vi "test12.2-AsyncMessageWithReply_Event.vi"(8 "error in (no error)":errorcluster, 11 "TestCase in":refnum<class "testcase-CSMGlobalLog.lvclass">) -> (0 "error out":errorcluster, 3 "TestCase out":refnum<class "testcase-CSMGlobalLog.lvclass">)   [LabVIEW 2017, in "testcase-CSMGlobalLog.lvclass"]
uses:
  testcase-CSMGlobalLog.lvclass
  testcase-CSMGlobalLog.lvclass/testcase-CSMGlobalLog.ctl
  src/user.lib/_NEVSTOP/Communicable State Machine(CSM)/_Support/Typedef/_CSM_GlobalLog_MSG.ctl
  src/user.lib/_NEVSTOP/Communicable State Machine(CSM)/_Support/Typedef/_CSM_Response Source Message.ctl
  src/user.lib/_NEVSTOP/Communicable State Machine(CSM)/_Support/Typedef/_CSM_GlobalLog_MSG_TYPE.ctl
  c0dc643a-0362-49fc-99f4-5251266ba5a0.vi
  src/user.lib/_NEVSTOP/Communicable State Machine(CSM)/_Support/GlobalEvent/GEvt-Generate with Rule Check.vi
  src/user.lib/_NEVSTOP/Communicable State Machine(CSM)/AdvanceAPI/CSM - Convert Error to Argument.vi
  src/user.lib/_NEVSTOP/Communicable State Machine(CSM)/_Support/GlobalEvent/Cache-GEvt Refs.vi
  src/user.lib/_NEVSTOP/Communicable State Machine(CSM)/AdvanceAPI/CSM - Make String Arguments Safe.vi
  src/user.lib/_NEVSTOP/Communicable State Machine(CSM)/_Support/ChangeFlag/FlagInstance-GEvt Refs.vi
  src/user.lib/_NEVSTOP/Communicable State Machine(CSM)/AdvanceAPI/CSM - Keywords.vi
  src/user.lib/_NEVSTOP/Communicable State Machine(CSM)/_Support/ChangeFlag/ChangeFlag-Read.vi
  src/user.lib/_NEVSTOP/Communicable State Machine(CSM)/_Support/ChangeFlag/ChangeFlagDB.vi
  src/user.lib/_NEVSTOP/Communicable State Machine(CSM)/_Support/GlobalEvent/FGV-GlobalEventRef(lvlibp).vi
  src/user.lib/_NEVSTOP/Communicable State Machine(CSM)/_Support/GlobalEvent/FGV-GlobalEventQueues(lvlibp).vi
  src/user.lib/_NEVSTOP/Communicable State Machine(CSM)/_Support/GlobalEvent/GEvt-Valid Subscribers.vi
  src/user.lib/_NEVSTOP/Communicable State Machine(CSM)/_Support/GlobalEvent/LogFilter/LogFilter - Check.vi
  src/user.lib/_NEVSTOP/Communicable State Machine(CSM)/_Support/GlobalEvent/LogFilter/LogFilter.lvclass
  <vilib>/addons/_JKI Toolkits/VI Tester/TestCase.llb/TestCase.lvclass
  src/user.lib/_NEVSTOP/Communicable State Machine(CSM)/Communicable State Machine.lvlib
  C:/Program Files (x86)/National Instruments/LabVIEW 2017/vi.lib/addons/_JKI Toolkits/VI Tester/TestCase.llb/TestCase.lvclass
panel:
  out "String cache each loop":string
  out "LoopCount":i32
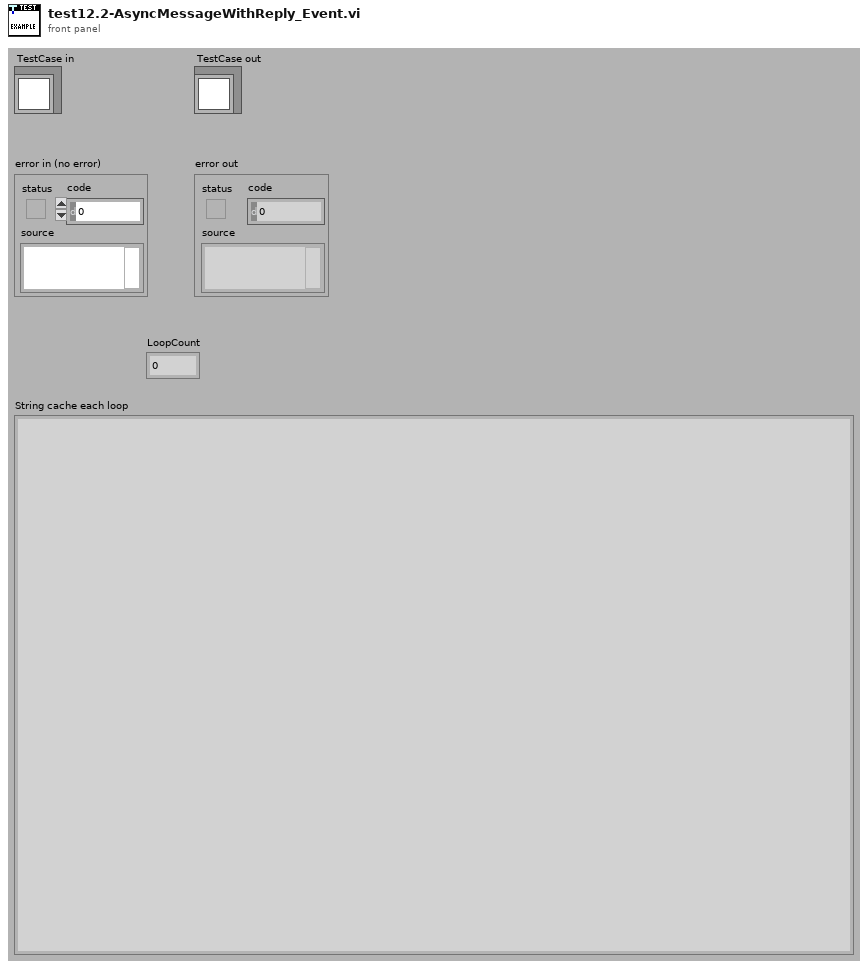
[diagram p1: front panel]
types:
  T1 = typedef "Communicable State Machine.lvlib/_CSM_GlobalLog_MSG.ctl" = cluster{"Name (\"\" to Use UUID)":string, "Current State":string, "Arguments":string, "Source Message":T2, "Source Module":string, "Complete(T)/Start(F)":bool, "LogType":T3, "Time Stamp":timestamp}
  T2 = typedef "Communicable State Machine.lvlib/_CSM_Response Source Message.ctl" = cluster{"‘State":string, "’Arguments":string, "’Error":errorcluster}
  T3 = typedef "Communicable State Machine.lvlib/_CSM_GlobalLog_MSG_TYPE.ctl" = enum16{"User Log", "State Change", "Status", "Interrupt", "Register", "Unregister", "Error Log", "Module Created", "Module Destroyed", "Async Message", "No-Rep Async Message", "Sync Message"}
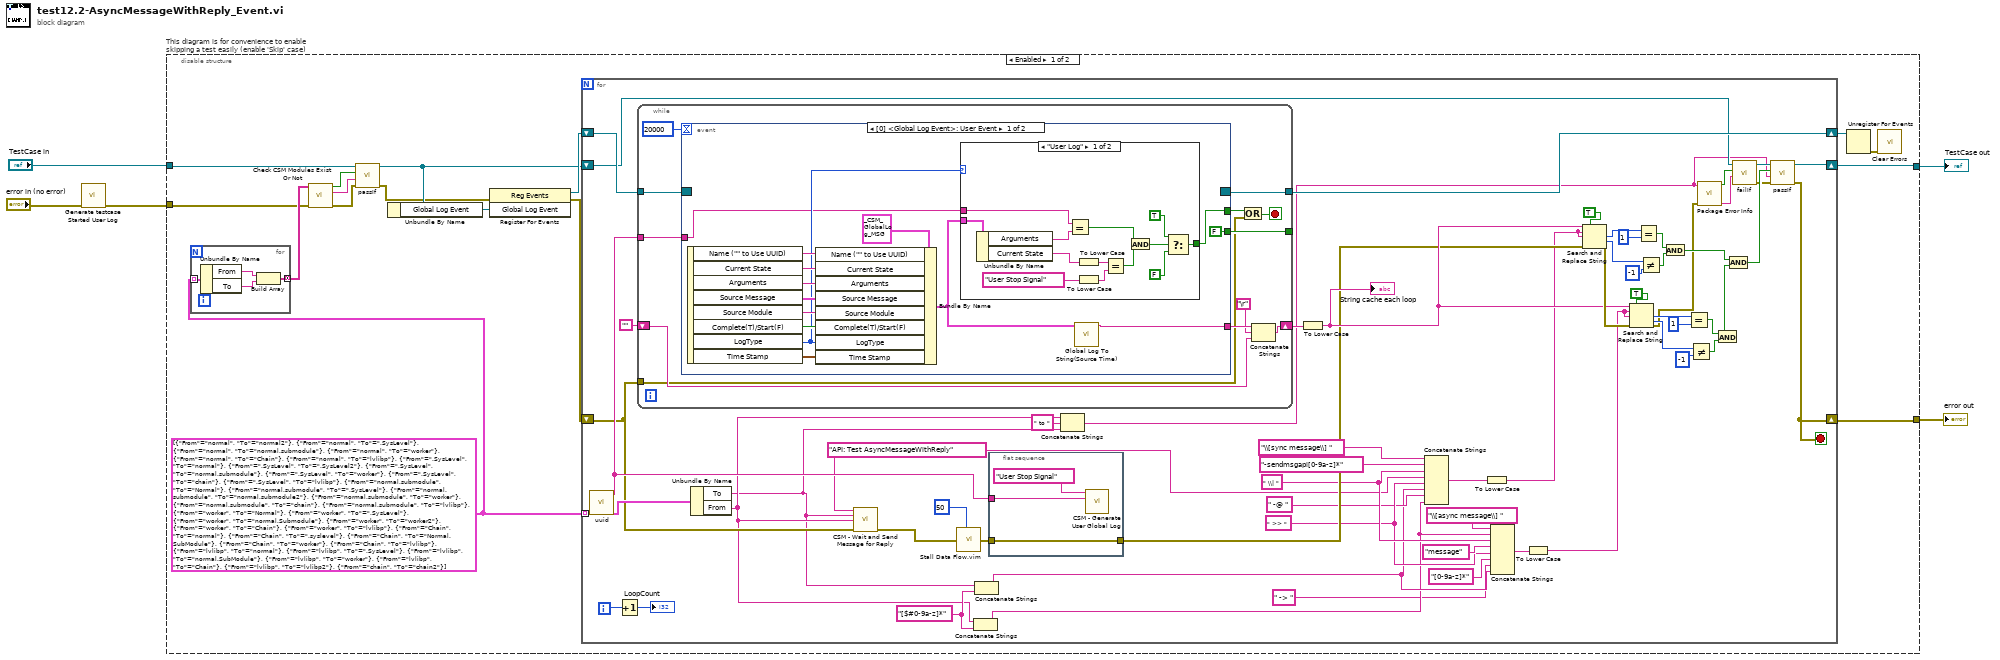
[diagram p0: block diagram]
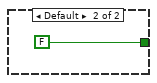
[diagram p2: hidden frame]
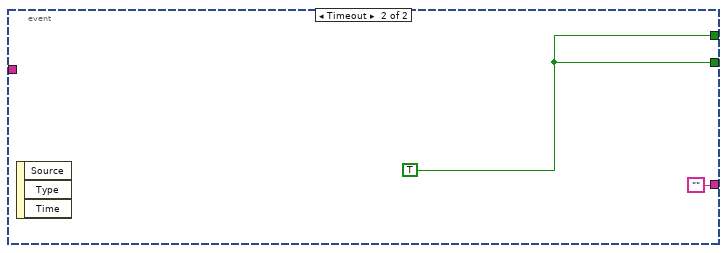
[diagram p3: hidden frame]
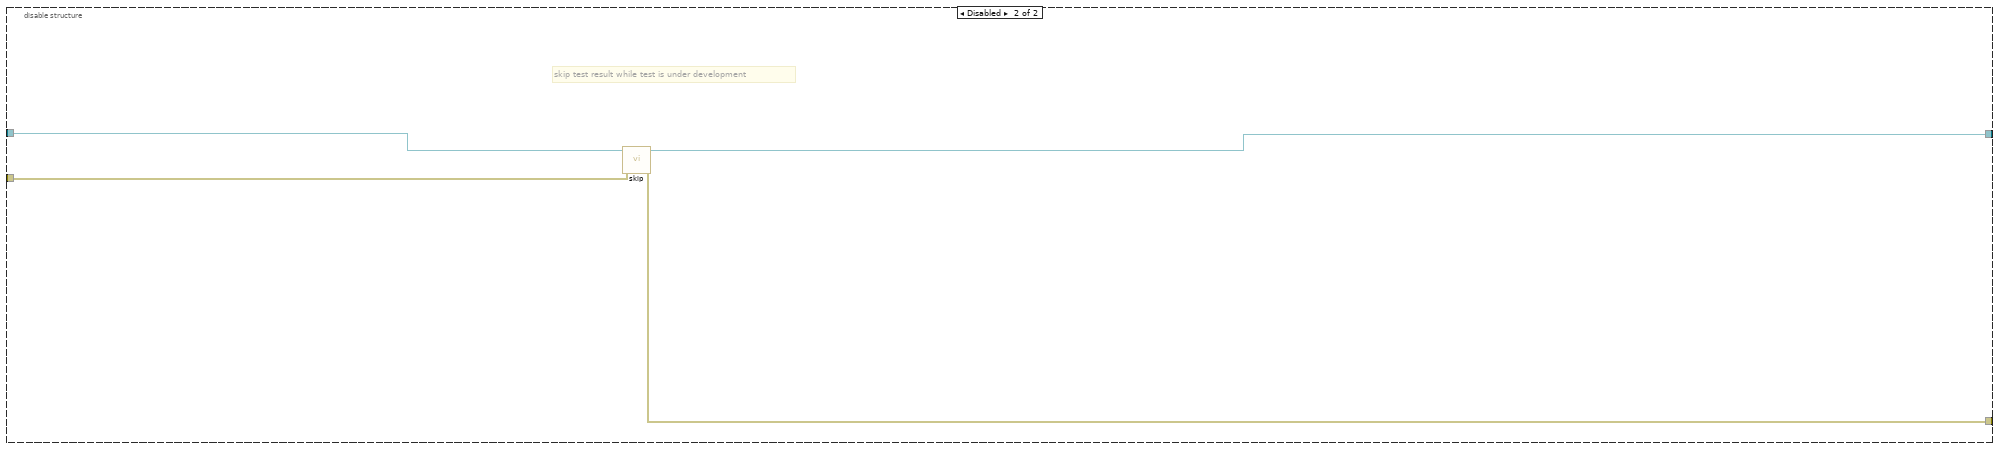
[diagram p4: hidden frame]
diagram:
  n1 = call "Generate testcase Started User Log.vi"("Error In"="error in (no error)") -> ("error out"=w1:errorcluster)  [unwired: 10 in]
  n2 = disable-structure "This diagram is for convenience to enable skipping a test easily (enable 'Skip' case)" shown="Enabled" {
    disable-tunnel: "TestCase in" -> [w9 w135]
    disable-tunnel: [w17 w133] -> w2
    disable-tunnel: [w16 w134] -> w4
    disable-tunnel: w1 -> [w10 w132]
    frame Enabled {
      w11 = cluster{"From":string, "To":string}[] [{"From"="normal", "To"="normal2"}, {"From"="normal", "To"=".SysLevel"}, {"From"="normal", "To"="normal.submodule"}, {"From"="normal", "To"="worker"}, {"From"="normal", "To"="Chain"}, {"From"="normal", "To"="lvlibp"}, {"From"=".SysLevel", "To"="normal"}, {"From"=".SysLevel", "To"=".SysLevel2"}, {"From"=".SysLevel", "To"="normal.submodule"}, {"From"=".SysLevel", "To"="worker"}, {"From"=".SysLevel", "To"="chain"}, {"From"=".SysLevel", "To"="lvlibp"}, {"From"="normal.submodule", "To"="Normal"}, {"From"="normal.submodule", "To"=".SysLevel"}, {"From"="normal.submodule", "To"="normal.submodule2"}, {"From"="normal.submodule", "To"="worker"}, {"From"="normal.submodule", "To"="chain"}, {"From"="normal.submodule", "To"="lvlibp"}, {"From"="worker", "To"="Normal"}, {"From"="worker", "To"=".SysLevel"}, {"From"="worker", "To"="normal.Submodule"}, {"From"="worker", "To"="worker2"}, {"From"="worker", "To"="Chain"}, {"From"="worker", "To"="lvlibp"}, {"From"="Chain", "To"="normal"}, {"From"="Chain", "To"=".syslevel"}, {"From"="Chain", "To"="Normal.SubModule"}, {"From"="Chain", "To"="worker"}, {"From"="Chain", "To"="lvlibp"}, {"From"="lvlibp", "To"="normal"}, {"From"="lvlibp", "To"=".SysLevel"}, {"From"="lvlibp", "To"="normal.SubModule"}, {"From"="lvlibp", "To"="worker"}, {"From"="lvlibp", "To"="Chain"}, {"From"="lvlibp", "To"="lvlibp2"}, {"From"="chain", "To"="chain2"}]
      n3 = for {
        tunnel: w11 -> [w25] mode=indexing
        tunnel: [w22] -> w14 mode=concatenating
        n4 = Unbundle By Name(w25) -> ("From"=w24:string, "To"=w23:string)
        n5 = Build Array(w24, w23) -> (w22:string[])
      }
      n6 = call "Check CSM Modules Exist Or Not.vi"("error in"=w10, "CSM names in"=w14) -> ("error out"=w12:errorcluster, "Debug string"=w13:string, "All Modules Exist?"=w15:bool)  [unwired: 7 in]
      n7 = call-dynamic "passIf.vi"("error in (no error)"=w12, "message (\"\")"=w13, "pass"=w15, "TestCase in"=w9) -> ("error out"=w7:errorcluster, "TestCase out"=w8:refnum<class "testcase-CSMGlobalLog.lvclass">)  [unwired: 6 in]
      n8 = Unbundle By Name(w8) -> ("Global Log Event"=w21:refnum<user-event>)
      n9 = register-events(error in=w7, w21) -> (reference out=w20:refnum<event-registration>, error out=w18:errorcluster)  [unwired: 1 in]
      n10 = for {
        shift-right: [w85] -> w19
        shift-left: w20 -> [w86]
        shift-right: [w82] -> w16
        shift-left: w18 -> [w36]
        tunnel: w11 -> [w63] mode=indexing
        shift-right: [w84] -> w17
        shift-left: w8 -> [w34]
        i -> [w60]
        stop <- w82 stop-if-true
        w41 = "[$#0-9a-z]*" ("string")
        w49 = " >> "
        w51 = " \\| "
        w44 = "API: Test AsyncMessageWithReply" ("State")
        n11 = call "uuid.vi"() -> ("UUID"=w61:string)  [unwired: 11 in]
        n12 = Increment(x=w60) -> (x+1=→"LoopCount":i32)
        n13 = while {
          tunnel: w86 -> [w101]
          tunnel: [w100] -> w85
          shift-right: [w92] -> w54
          shift-left: "" -> [w95]
          tunnel: w61 -> [w97]
          tunnel: [w96] -> _
          tunnel: w36 -> [w90]
          stop <- w91 stop-if-true
          n14 = event shown="[0] <Global Log Event>: User Event" {
            selector: w101 -> [_ _]
            dyn-events: [_ _] -> w100
            timeout: 20000 -> [_ _]
            tunnel: [w102 ""] -> w94
            tunnel: [w104 w131] -> w99
            tunnel: w97 -> [w105 _]
            tunnel: [FALSE ("Stop") w131] -> w96
            event User Event {
              n15 = event-data() -> ("Name (\"\" to Use UUID)"=w114:string, "Current State"=w113:string, "Arguments"=w112:string, "Source Message"=w111:T2, "Source Module"=w110:string, "Complete(T)/Start(F)"=w109:bool, "LogType"=w106:T3, "Time Stamp"=w108:timestamp)  [unwired: 1 in]
              n16 = Bundle By Name(cluster=T1 {"Name (\"\" to Use UUID)"="", "Current State"="", "Arguments"="", "Source Message"={"‘State"="", "’Arguments"="", "’Error"={"status"=FALSE, "code"=0, "source"=""}}, "Source Module"="", "Complete(T)/Start(F)"=FALSE, "LogType"=enum."State Change", "Time Stamp"=timestamp(0 s since 1904-01-01)} ("Cross CSM Data"), "Name (\"\" to Use UUID)"=w114, "Current State"=w113, "Arguments"=w112, "Source Message"=w111, "Source Module"=w110, "Complete(T)/Start(F)"=w109, "LogType"=w106, "Time Stamp"=w108) -> (w103:T1)
              n17 = case shown="\"User Log\"" w106 {
                tunnel: w103 -> [w128 _]
                tunnel: w105 -> [w127 _]
                tunnel: [w116 FALSE] -> w104
                frame "User Log" {
                  n18 = Unbundle By Name(w128) -> ("Arguments"=w126:string, "Current State"=w125:string)
                  n19 = Equal?(x=w127, y=w126) -> (x = y?=w120:bool)
                  n20 = To Lower Case(string=w125) -> (all lower case string=w124:string)
                  n21 = To Lower Case(string="User Stop Signal" ("Log")) -> (all lower case string=w122:string)
                  n22 = Equal?(x=w124, y=w122) -> (x = y?=w121:bool)
                  n23 = And(x=w120, y=w121) -> (x .and. y?=w119:bool)
                  n24 = Select(t=TRUE, s=w119, f=FALSE) -> (s? t:f=w116:bool)
                }
                frame Default {
                }
              }
              n25 = call "Global Log To String(Source Time).vi"("Log"=w103) -> ("Log String"=w102:string)  [unwired: 9 in]
            }
            event Timeout {
              w131 = TRUE ("Stop")
              n26 = event-data() -> ()  [unwired: 1 in, 3 out]
            }
          }
          n27 = Or(x=w99, y=w90) -> (x .or. y?=w91:bool)
          n28 = Concatenate Strings(w94, "\r", w95) -> (w92:string)
        }
        n29 = Unbundle By Name(w63) -> ("To"=w28:string, "From"=w29:string)
        n30 = call "CSM - Wait and Send Message for Reply.vi"("State"=w44, "Arguments (\"\")"=w28, "Target Module"=w29, "Error In (No Error)"=w36) -> ("error out"=w57:errorcluster)  [unwired: 8 in, 3 out]
        n31 = call "Stall Data Flow.vim"("value in"=w57, "milliseconds to wait"=u32 50) -> ("value out"=w62:errorcluster)  [unwired: 1 out]
        n32 = Concatenate Strings(w29, w41) -> (w39:string)
        n33 = Concatenate Strings(w28, w41) -> (w40:string)
        n34 = flat-sequence {
          tunnel: w61 -> [w88]
          tunnel: w62 -> [w87]
          tunnel: [w87] -> w55
          frame #0 {
            n35 = call "CSM - Generate User Global Log.vi"("Arguments"=w88, "Log"="User Stop Signal") -> ()  [unwired: 9 in, 1 out]
          }
        }
        n36 = Concatenate Strings(w29, " to " ("string"), w28) -> (w26:string)
        n37 = To Lower Case(string=w54) -> (all lower case string=w56:string)
        "String cache each loop" <- w56
        n38 = Concatenate Strings("\\[sync message\\] ", "-sendmsgapi[0-9a-z]*", w51, w44, w49, w40, " -@ ", w39) -> (w46:string)
        n39 = To Lower Case(string=w46) -> (all lower case string=w43:string)
        n40 = Concatenate Strings("\\[async message\\] " ("string"), w39, w51, "message", w49, "[0-9a-z]*", " -> ", w40) -> (w45:string)
        n41 = To Lower Case(string=w45) -> (all lower case string=w42:string)
        n42 = Search and Replace String(replace all?=TRUE ("replace all? (F)"), input string=w56, search string=w43, replace string=w43, error in=w55) -> (number of replacements=w71:i32, offset past replacement=w72:i32, error out=w79:errorcluster)  [unwired: 3 in, 1 out]
        n43 = Search and Replace String(replace all?=TRUE ("replace all? (F)"), input string=w56, search string=w42, replace string=w42, error in=w79) -> (number of replacements=w78:i32, offset past replacement=w77:i32, error out=w30:errorcluster)  [unwired: 3 in, 1 out]
        n44 = Equal?(x=w71, y=1) -> (x = y?=w73:bool)
        n45 = Not Equal?(x=w72, y=-1) -> (x != y?=w74:bool)
        n46 = And(x=w73, y=w74) -> (x .and. y?=w81:bool)
        n47 = Equal?(x=w78, y=1) -> (x = y?=w76:bool)
        n48 = Not Equal?(x=w77, y=-1) -> (x != y?=w75:bool)
        n49 = call "Package Error Info.vi"("error in"=w30, "String in"=w26) -> ("packed error info out"=w31:string, "error status"=w35:bool)  [unwired: 8 in]
        n50 = And(x=w76, y=w75) -> (x .and. y?=w80:bool)
        n51 = And(x=w81, y=w80) -> (x .and. y?=w59:bool)
        n52 = call-dynamic "failIf.vi"("message (\"\")"=w31, "fail"=w35, "TestCase in"=w34) -> ("error out"=w32:errorcluster, "TestCase out"=w33:refnum<class "testcase-CSMGlobalLog.lvclass">)  [unwired: 7 in]
        n53 = call-dynamic "passIf.vi"("error in (no error)"=w32, "message (\"\")"=w26, "pass"=w59, "TestCase in"=w33) -> ("error out"=w82:errorcluster, "TestCase out"=w84:refnum<class "testcase-CSMGlobalLog.lvclass">)  [unwired: 6 in]
      }
      n54 = Unregister For Events(event registration refnum=w19) -> (error out=w6:errorcluster)  [unwired: 1 in]
      n55 = call <vilib>:"Clear Errors.vi"("error in (no error)"=w6) -> ()  [unwired: 5 in, 2 out]
    }
    frame Disabled {
      # "skip test result while test is under development"
      n56 = call <vilib>:"skip.vi"("error in (no error)"=w132, "TestCase in"=w135) -> ("error out"=w134:errorcluster, "TestCase out"=w133:refnum<class "testcase-CSMGlobalLog.lvclass">)  [unwired: 8 in]
    }
  }
  "error out" <- w4
  "TestCase out" <- w2
